vi "test_tcpclient.vi"() -> ()   [LabVIEW 2019]
panel:
  out "에러 출력":errorcluster
  out "길이":i32
  out "데이터 출력":string
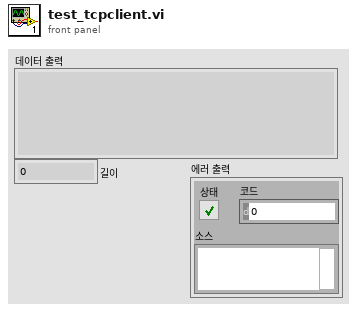
[diagram p1: front panel]
types:
  T1 = enum16{"Standard", "Buffered", "CRLF", "Immediate"}
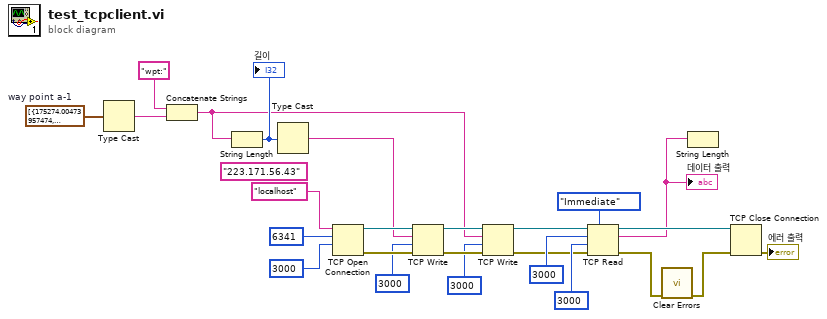
[diagram p0: block diagram]
diagram:
  (unwired) "223.171.56.43" ("Machine")
  w12 = cluster{"X":dbl, "Y":dbl}[] [{"X"=175274.00473957474, "Y"=530129.5157438602}, {"X"=175273.9994878598, "Y"=530129.5122022912}, {"X"=175273.88617325024, "Y"=530129.3515401008}, {"X"=175272.68065750896, "Y"=530127.4900123067}, {"X"=175272.6737370609, "Y"=530127.4862059783}, {"X"=175272.6643477536, "Y"=530127.4868430574}, {"X"=175272.65941880862, "Y"=530127.4861129179}, {"X"=175272.65828264618, "Y"=530127.4796280419}, {"X"=175272.65754210684, "Y"=530127.4685405197}, {"X"=175272.65886747447, "Y"=530127.4575323473}, {"X"=175275.24952781235, "Y"=530130.7235086206}, {"X"=175275.72679590562, "Y"=530131.2911066092}, {"X"=175276.22262929002, "Y"=530131.8883650973}, {"X"=175276.73046744007, "Y"=530132.5103790438}, {"X"=175277.2160084758, "Y"=530133.111474839}, {"X"=175277.7228783223, "Y"=530133.7379877474}, {"X"=175278.23467314534, "Y"=530134.3806933991}, {"X"=175278.74720273982, "Y"=530135.0409537714}, {"X"=175279.23987504462, "Y"=530135.6864052094}, {"X"=175280.91154517294, "Y"=530137.9295182931}, {"X"=175281.1794743994, "Y"=530138.2947289064}, {"X"=175281.44680856468, "Y"=530138.6510235704}, {"X"=175281.72463026966, "Y"=530139.0159308233}, {"X"=175282.0015102056, "Y"=530139.3688022257}, {"X"=175282.27945698082, "Y"=530139.7259944954}, {"X"=175282.55852373713, "Y"=530140.077914963}, {"X"=175282.8311483772, "Y"=530140.4203407691}, {"X"=175283.1033063822, "Y"=530140.7571409787}, {"X"=175283.37576432535, "Y"=530141.0959280683}, {"X"=175283.65336961742, "Y"=530141.4368242207}, {"X"=175283.92779126446, "Y"=530141.7740950054}, {"X"=175284.20385452232, "Y"=530142.1228424397}, {"X"=175284.47496994474, "Y"=530142.4665701878}, {"X"=175284.74596157094, "Y"=530142.8094792332}, {"X"=175285.0186950549, "Y"=530143.1588214315}, {"X"=175285.29130561682, "Y"=530143.5103371057}, {"X"=175285.56377946716, "Y"=530143.8635579381}, {"X"=175285.83036446967, "Y"=530144.2140548322}, {"X"=175286.10275126458, "Y"=530144.5741004624}, {"X"=175286.36828605848, "Y"=530144.9232298034}, {"X"=175286.63513163378, "Y"=530145.2764972708}, {"X"=175286.90739945296, "Y"=530145.6370704629}, {"X"=175287.1797670756, "Y"=530145.994256079}, {"X"=175287.4453014945, "Y"=530146.342989234}, {"X"=175287.70847312824, "Y"=530146.6934008283}, {"X"=175287.96834295726, "Y"=530147.0397678753}, {"X"=175288.21933206188, "Y"=530147.3826218339}, {"X"=175288.48230602973, "Y"=530147.73750566}, {"X"=175288.72661496594, "Y"=530148.0667469767}, {"X"=175288.97248932836, "Y"=530148.3963732349}, {"X"=175289.20325854485, "Y"=530148.6997193932}, {"X"=175289.4533325028, "Y"=530149.0263799197}, {"X"=175289.7170391103, "Y"=530149.3732351185}, {"X"=175289.94705338945, "Y"=530149.6807133132}, {"X"=175290.20929376624, "Y"=530150.0313974353}, {"X"=175290.44099765085, "Y"=530150.3384233768}, {"X"=175290.69107477734, "Y"=530150.6691870798}, {"X"=175290.93328572533, "Y"=530150.9923448646}, {"X"=175291.17306334805, "Y"=530151.3085965351}, {"X"=175291.42890964248, "Y"=530151.6447770832}, {"X"=175291.65563403358, "Y"=530151.9375893783}, {"X"=175291.89275191838, "Y"=530152.2404695762}, {"X"=175292.13425833316, "Y"=530152.5476597142}, {"X"=175292.38933595005, "Y"=530152.872240096}, {"X"=175292.63073491893, "Y"=530153.1751564976}, {"X"=175292.86438353983, "Y"=530153.4646986987}, {"X"=175293.08456251005, "Y"=530153.7373553545}, {"X"=175293.31933611992, "Y"=530154.0296189471}, {"X"=175293.5669353489, "Y"=530154.3429552813}, {"X"=175293.79013514795, "Y"=530154.6346082591}, {"X"=175293.99919699648, "Y"=530154.91043425}, {"X"=175294.23494612498, "Y"=530155.2225936522}, {"X"=175294.4618142799, "Y"=530155.528153441}, {"X"=175294.68670046306, "Y"=530155.8245694136}, {"X"=175294.8932319965, "Y"=530156.1005460762}, {"X"=175295.11416787718, "Y"=530156.3949848645}, {"X"=175295.3423867288, "Y"=530156.7029191155}, {"X"=175295.54093274107, "Y"=530156.9698773636}, {"X"=175295.77252229722, "Y"=530157.2770136676}, {"X"=175295.99228581943, "Y"=530157.568919915}, {"X"=175296.2108791497, "Y"=530157.857811919}, {"X"=175296.43384412082, "Y"=530158.1500960607}, {"X"=175296.65676498265, "Y"=530158.4451449964}, {"X"=175296.87656675442, "Y"=530158.733828123}, {"X"=175297.09878029334, "Y"=530159.0242344007}, {"X"=175297.3209100406, "Y"=530159.3192634964}, {"X"=175297.53946949937, "Y"=530159.61111341}, {"X"=175297.75729462548, "Y"=530159.9050631305}, {"X"=175297.97451755032, "Y"=530160.1915685921}, {"X"=175298.19257092883, "Y"=530160.4863322874}, {"X"=175298.40867646263, "Y"=530160.7769064768}, {"X"=175298.62256852756, "Y"=530161.0666281783}, {"X"=175298.83417822816, "Y"=530161.3513644824}, {"X"=175299.04778942713, "Y"=530161.6437706635}, {"X"=175299.47700209834, "Y"=530162.2207681962}, {"X"=175299.6962516632, "Y"=530162.5195904814}, {"X"=175299.91551021635, "Y"=530162.8160642846}, {"X"=175300.12963692454, "Y"=530163.1102869193}, {"X"=175300.34073252836, "Y"=530163.3991423576}, {"X"=175300.54502428067, "Y"=530163.6795729806}, {"X"=175300.7577223589, "Y"=530163.9708631652}, {"X"=175301.62616935943, "Y"=530165.1216823726}, {"X"=175302.5254593493, "Y"=530166.2863037863}, {"X"=175303.18527895535, "Y"=530167.1454968242}, {"X"=175303.62342696637, "Y"=530167.7159166778}, {"X"=175310.16097941765, "Y"=530176.5582115706}, {"X"=175311.60845001024, "Y"=530178.4564093163}, {"X"=175311.86030556855, "Y"=530178.7900606951}, {"X"=175312.11498075575, "Y"=530179.126174304}, {"X"=175312.62935982816, "Y"=530179.7996497159}, {"X"=175313.1375920335, "Y"=530180.4658226775}, {"X"=175313.3990189692, "Y"=530180.8068619235}, {"X"=175313.65881998377, "Y"=530181.146539741}, {"X"=175313.9177177645, "Y"=530181.4836165035}, {"X"=175314.17415214767, "Y"=530181.8221921967}, {"X"=175314.4395212584, "Y"=530182.1661021416}, {"X"=175314.7023115845, "Y"=530182.5087333805}, {"X"=175314.96900353231, "Y"=530182.8527781678}, {"X"=175315.23369983808, "Y"=530183.1956435259}, {"X"=175315.50157477424, "Y"=530183.5455604322}, {"X"=175315.77181018525, "Y"=530183.8960341865}, {"X"=175316.04542567665, "Y"=530184.247385859}, {"X"=175316.31955375904, "Y"=530184.6010511945}, {"X"=175316.84903058026, "Y"=530185.2820837225}, {"X"=175317.38129618068, "Y"=530185.9581514191}, {"X"=175317.91280706186, "Y"=530186.6327397156}, {"X"=175318.182062935, "Y"=530186.9719269531}, {"X"=175318.4552795316, "Y"=530187.3193476506}, {"X"=175319.0014159784, "Y"=530188.0142099282}, {"X"=175319.27483774978, "Y"=530188.3555402486}, {"X"=175319.5492389786, "Y"=530188.6974037511}, {"X"=175319.82539301965, "Y"=530189.0371189493}, {"X"=175320.09826249993, "Y"=530189.381323244}, {"X"=175320.37226519384, "Y"=530189.7271334985}, {"X"=175320.64393428696, "Y"=530190.0701027507}, {"X"=175320.9165769911, "Y"=530190.4185252064}, {"X"=175321.19328325742, "Y"=530190.7740132491}, {"X"=175321.45659139234, "Y"=530191.1140005968}, {"X"=175321.72941233087, "Y"=530191.461311584}, {"X"=175321.95251283867, "Y"=530191.7470001135}, {"X"=175322.16532464704, "Y"=530192.0220943327}, {"X"=175322.37067224752, "Y"=530192.2834971666}, {"X"=175322.56229437568, "Y"=530192.525027423}, {"X"=175322.73990554007, "Y"=530192.7495959902}, {"X"=175322.91422045446, "Y"=530192.9731865155}, {"X"=175323.08738154572, "Y"=530193.1905985337}, {"X"=175323.26548979027, "Y"=530193.4137283771}, {"X"=175323.43727148935, "Y"=530193.6328725251}, {"X"=175323.6096645412, "Y"=530193.8490726349}, {"X"=175323.80699074292, "Y"=530194.0964960849}, {"X"=175324.05614273442, "Y"=530194.4061107116}, {"X"=175324.31111888157, "Y"=530194.7286735323}, {"X"=175324.56704112957, "Y"=530195.0488684587}, {"X"=175324.83578187227, "Y"=530195.3871728731}, {"X"=175325.10834637488, "Y"=530195.7293249926}, {"X"=175325.38945439694, "Y"=530196.0823263065}, {"X"=175325.6722181846, "Y"=530196.4354126442}, {"X"=175325.95672967637, "Y"=530196.789425005}, {"X"=175326.24457830185, "Y"=530197.1504762445}, {"X"=175326.5286249899, "Y"=530197.506083755}, {"X"=175326.8080508342, "Y"=530197.8612032551}, {"X"=175327.0941640386, "Y"=530198.2291274525}, {"X"=175327.37333938808, "Y"=530198.5921299302}, {"X"=175327.65607127667, "Y"=530198.9641828123}, {"X"=175327.9397818841, "Y"=530199.334716748}, {"X"=175328.220501643, "Y"=530199.707514753}, {"X"=175328.5049111398, "Y"=530200.0795682647}, {"X"=175328.7949704538, "Y"=530200.4580267589}, {"X"=175329.07385205853, "Y"=530200.8277980806}, {"X"=175329.36379046313, "Y"=530201.2178327836}, {"X"=175329.66436532678, "Y"=530201.6225661638}, {"X"=175329.95547737126, "Y"=530202.0138116102}, {"X"=175330.25295598558, "Y"=530202.41901918}, {"X"=175330.53956022885, "Y"=530202.8108706116}, {"X"=175330.8419255085, "Y"=530203.2223300473}, {"X"=175331.13195201478, "Y"=530203.6179626812}, {"X"=175331.41571912347, "Y"=530204.010755906}, {"X"=175331.69713162916, "Y"=530204.4019945143}, {"X"=175331.98958687438, "Y"=530204.8024301422}, {"X"=175332.29121012747, "Y"=530205.2164278494}, {"X"=175332.5883215296, "Y"=530205.6155401273}, {"X"=175332.88285866773, "Y"=530206.0119009}, {"X"=175333.19089243043, "Y"=530206.4178487876}, {"X"=175333.49203705165, "Y"=530206.816168969}, {"X"=175333.79303850673, "Y"=530207.2110079534}, {"X"=175334.0893020318, "Y"=530207.5938922067}, {"X"=175334.3892063653, "Y"=530207.9855713523}, {"X"=175334.6769313669, "Y"=530208.3671245654}, {"X"=175334.95773330683, "Y"=530208.7361556918}, {"X"=175335.2323387888, "Y"=530209.0990575975}, {"X"=175335.51306748565, "Y"=530209.4603920867}, {"X"=175335.795338003, "Y"=530209.8291292372}, {"X"=175336.075867931, "Y"=530210.1873578326}, {"X"=175336.3589926412, "Y"=530210.5538095022}, {"X"=175336.63876707532, "Y"=530210.9195896094}, {"X"=175336.91411793797, "Y"=530211.2847901087}, {"X"=175337.18312003254, "Y"=530211.6465776593}, {"X"=175337.45269431596, "Y"=530212.0062625683}, {"X"=175337.7209553494, "Y"=530212.3690822715}, {"X"=175337.98944422093, "Y"=530212.7334773109}, {"X"=175338.25587926744, "Y"=530213.0979849639}, {"X"=175338.52868281276, "Y"=530213.4681063772}, {"X"=175338.8270715183, "Y"=530213.8710219278}, {"X"=175339.09987210427, "Y"=530214.2401578118}, {"X"=175339.36014116515, "Y"=530214.5890679677}, {"X"=175339.64015941726, "Y"=530214.9682290286}, {"X"=175339.91455805866, "Y"=530215.3392247901}, {"X"=175340.19204513606, "Y"=530215.716735207}, {"X"=175340.47255665058, "Y"=530216.0988848016}, {"X"=175340.7614513212, "Y"=530216.4867809507}, {"X"=175341.04350502143, "Y"=530216.8716629283}, {"X"=175341.33658991486, "Y"=530217.2774543162}, {"X"=175341.64410756333, "Y"=530217.7099119138}, {"X"=175341.923443017, "Y"=530218.1057118566}, {"X"=175342.22936364054, "Y"=530218.5355027524}, {"X"=175342.55279432627, "Y"=530218.9959007761}, {"X"=175342.853771716, "Y"=530219.4237218449}, {"X"=175343.1555258112, "Y"=530219.8539135159}, {"X"=175343.45287598448, "Y"=530220.2793768641}, {"X"=175343.75118908664, "Y"=530220.7039772415}, {"X"=175344.02648011563, "Y"=530221.0926561153}, {"X"=175344.31951030123, "Y"=530221.513938076}, {"X"=175344.61748993694, "Y"=530221.9456370183}, {"X"=175344.9215387921, "Y"=530222.3808929314}, {"X"=175345.2398094967, "Y"=530222.8343840825}, {"X"=175345.54070788863, "Y"=530223.261942445}, {"X"=175345.84672666568, "Y"=530223.6909019012}, {"X"=175346.14135953155, "Y"=530224.0964236386}, {"X"=175346.4818114266, "Y"=530224.5620700925}, {"X"=175346.79941728554, "Y"=530224.9956179837}, {"X"=175347.12591049456, "Y"=530225.4394857899}, {"X"=175347.44286325248, "Y"=530225.866352058}, {"X"=175347.7636738763, "Y"=530226.3017351214}, {"X"=175348.0793182589, "Y"=530226.7285975026}, {"X"=175348.3978399274, "Y"=530227.1606688595}, {"X"=175348.71413229345, "Y"=530227.5958266628}, {"X"=175349.03568725986, "Y"=530228.0346559128}, {"X"=175349.35136932984, "Y"=530228.4656335876}, {"X"=175349.63429763477, "Y"=530228.8502990768}, {"X"=175350.31202571455, "Y"=530229.7610748007}, {"X"=175350.9657620107, "Y"=530230.6222051637}, {"X"=175351.30501294706, "Y"=530231.0718611733}, {"X"=175352.98191093397, "Y"=530233.2849793285}, {"X"=175354.325094944, "Y"=530235.0392812236}, {"X"=175356.5139735839, "Y"=530237.9021652578}, {"X"=175357.11627366152, "Y"=530238.6805678556}, {"X"=175357.40969987572, "Y"=530239.059631174}, {"X"=175357.9977159878, "Y"=530239.8222138252}, {"X"=175358.58175825854, "Y"=530240.5853587184}, {"X"=175358.8800216713, "Y"=530240.9707595569}, {"X"=175359.17089952106, "Y"=530241.3456795723}, {"X"=175359.45570521321, "Y"=530241.7094456495}, {"X"=175359.7556257851, "Y"=530242.08400608}, {"X"=175360.0654265399, "Y"=530242.4592355064}, {"X"=175360.37610858618, "Y"=530242.8335511507}, {"X"=175360.6766469507, "Y"=530243.1926461258}, {"X"=175360.9757493711, "Y"=530243.5442038479}, {"X"=175361.28149900775, "Y"=530243.8940705459}, {"X"=175361.58179288538, "Y"=530244.242366232}, {"X"=175361.8795235083, "Y"=530244.5943442258}, {"X"=175362.1701690775, "Y"=530244.9335109157}, {"X"=175362.47002807373, "Y"=530245.2797391374}, {"X"=175362.75999962015, "Y"=530245.619241903}, {"X"=175363.04848654536, "Y"=530245.9575326451}, {"X"=175363.32893681235, "Y"=530246.291935935}, {"X"=175363.5833795738, "Y"=530246.5938537038}, {"X"=175363.8139917913, "Y"=530246.8664914699}, {"X"=175364.051439322, "Y"=530247.149266535}, {"X"=175364.27875054546, "Y"=530247.4193158604}, {"X"=175364.48140306285, "Y"=530247.6667112568}, {"X"=175364.68130373914, "Y"=530247.9081936695}, {"X"=175364.87212307978, "Y"=530248.1351448188}, {"X"=175365.05830122996, "Y"=530248.3405561815}, {"X"=175365.24934642285, "Y"=530248.5335349937}, {"X"=175365.4586938402, "Y"=530248.7211780654}, {"X"=175365.68035351747, "Y"=530248.885941745}, {"X"=175365.90327231257, "Y"=530249.0346165324}, {"X"=175366.13637149328, "Y"=530249.1652904893}, {"X"=175366.37079705653, "Y"=530249.2714382051}, {"X"=175366.61827390923, "Y"=530249.3659272505}, {"X"=175366.86756814134, "Y"=530249.4425965978}, {"X"=175367.11207690288, "Y"=530249.5058751716}, {"X"=175367.3567533101, "Y"=530249.5650245816}, {"X"=175367.62133496685, "Y"=530249.629879967}, {"X"=175367.86905430927, "Y"=530249.6933355606}, {"X"=175368.1517549946, "Y"=530249.7661407787}, {"X"=175368.41413817744, "Y"=530249.8400324802}, {"X"=175368.67676292398, "Y"=530249.9249654686}, {"X"=175368.95770089532, "Y"=530250.0176168601}, {"X"=175369.22670276524, "Y"=530250.1089982273}, {"X"=175369.50063303096, "Y"=530250.2033583766}, {"X"=175369.77402096745, "Y"=530250.2964393551}, {"X"=175370.0421101817, "Y"=530250.3874249985}, {"X"=175370.29664589485, "Y"=530250.4816636177}, {"X"=175370.53368479141, "Y"=530250.5680904333}, {"X"=175370.78877829644, "Y"=530250.6574362741}, {"X"=175371.04713739155, "Y"=530250.7475893599}, {"X"=175371.29533503368, "Y"=530250.8288002849}, {"X"=175371.55924210517, "Y"=530250.9034323096}, {"X"=175371.81141736405, "Y"=530250.9751788629}, {"X"=175372.05235837863, "Y"=530251.0394492042}, {"X"=175372.29207432698, "Y"=530251.0964913194}, {"X"=175372.54753447103, "Y"=530251.1479322227}, {"X"=175372.80985884863, "Y"=530251.1964750472}, {"X"=175373.0779618144, "Y"=530251.240423805}, {"X"=175373.34660774906, "Y"=530251.2834664334}, {"X"=175373.6152436773, "Y"=530251.3234125947}, {"X"=175373.88194546604, "Y"=530251.3601902636}, {"X"=175374.1938507625, "Y"=530251.4006926748}, {"X"=175374.51872925175, "Y"=530251.4433166765}, {"X"=175374.79900635238, "Y"=530251.482146475}, {"X"=175375.13868270424, "Y"=530251.5259788403}, {"X"=175375.45358824547, "Y"=530251.5683248173}, {"X"=175375.82978955292, "Y"=530251.6141916682}, {"X"=175376.17793499245, "Y"=530251.6580746012}, {"X"=175376.5139992762, "Y"=530251.7055702066}, {"X"=175376.87018973782, "Y"=530251.7555936353}, {"X"=175377.24026591453, "Y"=530251.8047892973}, {"X"=175377.59636930356, "Y"=530251.8604399993}, {"X"=175377.96688510012, "Y"=530251.9082270975}, {"X"=175378.35741249754, "Y"=530251.9509165223}, {"X"=175378.67374899556, "Y"=530251.9738647275}, {"X"=175379.00524160772, "Y"=530251.975895192}, {"X"=175379.35247739623, "Y"=530251.9689682503}, {"X"=175379.7125607502, "Y"=530251.9581977867}, {"X"=175380.0933729456, "Y"=530251.9500654789}, {"X"=175380.45119064956, "Y"=530251.9423638212}, {"X"=175380.79150680685, "Y"=530251.9408800876}, {"X"=175381.1301878372, "Y"=530251.9403068274}, {"X"=175381.47107652182, "Y"=530251.9410356049}, {"X"=175381.81160542736, "Y"=530251.941713292}, {"X"=175382.1583224557, "Y"=530251.9436135975}, {"X"=175382.50416204456, "Y"=530251.9471435535}, {"X"=175382.85047314703, "Y"=530251.951369127}, {"X"=175383.20556531035, "Y"=530251.9538985235}, {"X"=175383.55283039506, "Y"=530251.9560181338}, {"X"=175383.89244492707, "Y"=530251.9614254886}, {"X"=175384.2278018331, "Y"=530251.9786764916}, {"X"=175384.56469375637, "Y"=530252.0103555985}, {"X"=175384.90371252302, "Y"=530252.051392338}, {"X"=175385.24706478935, "Y"=530252.099438415}, {"X"=175385.58792804737, "Y"=530252.1459935226}, {"X"=175385.9193890007, "Y"=530252.1932400188}, {"X"=175386.2604837821, "Y"=530252.2369021791}, {"X"=175386.5911148225, "Y"=530252.2775530318}, {"X"=175386.9222903062, "Y"=530252.3006465423}, {"X"=175387.28229401182, "Y"=530252.2929121043}, {"X"=175387.62466421502, "Y"=530252.2799721844}, {"X"=175387.93027813133, "Y"=530252.2646488417}, {"X"=175388.2409991896, "Y"=530252.2450208705}, {"X"=175388.56240209253, "Y"=530252.220650116}, {"X"=175388.92052526696, "Y"=530252.190338978}, {"X"=175389.23687064392, "Y"=530252.1678687864}, {"X"=175389.5753376039, "Y"=530252.1406143736}, {"X"=175389.8778530315, "Y"=530252.1153481143}, {"X"=175390.22718472683, "Y"=530252.089512334}, {"X"=175390.5630890984, "Y"=530252.0655584557}, {"X"=175390.8979634547, "Y"=530252.0428584341}, {"X"=175391.22960317053, "Y"=530252.0226429336}, {"X"=175391.55867739816, "Y"=530252.0038422944}, {"X"=175391.87951033696, "Y"=530251.9907639447}, {"X"=175392.2046095326, "Y"=530251.9799060859}, {"X"=175392.52962813876, "Y"=530251.968753254}, {"X"=175392.83001022547, "Y"=530251.9584021192}, {"X"=175393.14728301077, "Y"=530251.9506727168}, {"X"=175393.49708130673, "Y"=530251.9374026364}, {"X"=175393.82750725327, "Y"=530251.9267311599}, {"X"=175394.17059054173, "Y"=530251.9137949592}, {"X"=175394.4962388502, "Y"=530251.9011054165}, {"X"=175394.83817748734, "Y"=530251.8892968993}, {"X"=175395.1707083754, "Y"=530251.8805415569}, {"X"=175395.50018190366, "Y"=530251.874615377}, {"X"=175395.826819296, "Y"=530251.8750570489}, {"X"=175396.1583653206, "Y"=530251.8756751856}, {"X"=175396.5042830234, "Y"=530251.877458572}, {"X"=175396.8405475861, "Y"=530251.8822858657}, {"X"=175397.18239753207, "Y"=530251.8884995996}, {"X"=175397.50686157987, "Y"=530251.8956867978}, {"X"=175397.81604317346, "Y"=530251.9040510306}, {"X"=175398.4295024424, "Y"=530251.9020373435}, {"X"=175398.70534019003, "Y"=530251.8834735376}, {"X"=175398.99656782713, "Y"=530251.8608079262}, {"X"=175399.30757322672, "Y"=530251.8321375054}, {"X"=175399.6049048782, "Y"=530251.8016771716}, {"X"=175399.93269610187, "Y"=530251.7652727236}, {"X"=175400.25263059515, "Y"=530251.7277116233}, {"X"=175400.58998456638, "Y"=530251.686740851}, {"X"=175400.9279063112, "Y"=530251.6406464219}, {"X"=175401.27526716323, "Y"=530251.5958327602}, {"X"=175401.61223600793, "Y"=530251.5582338065}, {"X"=175401.9462553822, "Y"=530251.5348464095}, {"X"=175402.2982480789, "Y"=530251.5204725924}, {"X"=175402.64419659323, "Y"=530251.5128534149}, {"X"=175402.98677064007, "Y"=530251.5041509671}, {"X"=175403.32783964058, "Y"=530251.4963164325}, {"X"=175403.6796434534, "Y"=530251.4906012388}, {"X"=175404.0374824952, "Y"=530251.485324459}, {"X"=175404.73283554547, "Y"=530251.497987947}, {"X"=175405.44333194202, "Y"=530251.526324773}, {"X"=175405.78273774288, "Y"=530251.5408744316}, {"X"=175406.13260808703, "Y"=530251.5560026348}, {"X"=175406.84007820534, "Y"=530251.584189772}, {"X"=175407.21819518215, "Y"=530251.6017188046}, {"X"=175407.61685593953, "Y"=530251.6222140131}, {"X"=175408.01630098786, "Y"=530251.6416325923}, {"X"=175408.41382776093, "Y"=530251.6614641503}, {"X"=175408.80551302017, "Y"=530251.6828744787}, {"X"=175409.18886973435, "Y"=530251.7068475684}, {"X"=175409.5831748973, "Y"=530251.7272757728}, {"X"=175409.97421534616, "Y"=530251.7471941827}, {"X"=175410.3724366284, "Y"=530251.7664466639}, {"X"=175412.859882497, "Y"=530251.8016303764}, {"X"=175413.2918917442, "Y"=530251.7949316904}, {"X"=175413.71308979805, "Y"=530251.7872492936}, {"X"=175414.12900935306, "Y"=530251.7753028244}, {"X"=175415.85854146598, "Y"=530251.6858203384}, {"X"=175416.29044020732, "Y"=530251.6547917974}, {"X"=175417.58223410405, "Y"=530251.5570219693}, {"X"=175418.0143192921, "Y"=530251.5240274081}, {"X"=175419.74071979214, "Y"=530251.3542399728}, {"X"=175420.58187408207, "Y"=530251.2210568525}, {"X"=175421.8569027836, "Y"=530251.0132566964}, {"X"=175430.4214667419, "Y"=530249.9058980814}, {"X"=175434.9886332713, "Y"=530249.0412887661}, {"X"=175439.17077453557, "Y"=530248.2399495235}, {"X"=175440.32554478582, "Y"=530247.9882953187}, {"X"=175440.70893072494, "Y"=530247.8973494029}, {"X"=175441.44425972813, "Y"=530247.708410251}, {"X"=175442.51074655657, "Y"=530247.4062529192}, {"X"=175443.58120099697, "Y"=530247.1029309275}, {"X"=175444.74799694892, "Y"=530246.7786050664}, {"X"=175445.52227258962, "Y"=530246.5656788277}, {"X"=175445.89519918812, "Y"=530246.4617108132}, {"X"=175446.64006663952, "Y"=530246.2710016328}, {"X"=175447.56398738606, "Y"=530246.0934468561}, {"X"=175447.8627750396, "Y"=530246.0492128325}, {"X"=175448.4682387152, "Y"=530245.9726726192}, {"X"=175448.7696215642, "Y"=530245.9320069747}, {"X"=175449.06859093998, "Y"=530245.8998832443}, {"X"=175449.67792215856, "Y"=530245.847847441}, {"X"=175450.0131588634, "Y"=530245.8223230243}, {"X"=175450.34109198756, "Y"=530245.7966913233}, {"X"=175450.6775091883, "Y"=530245.772286645}, {"X"=175451.00768058727, "Y"=530245.748732713}, {"X"=175451.659518, "Y"=530245.7100337361}, {"X"=175452.61561360906, "Y"=530245.6690087137}, {"X"=175453.24432312453, "Y"=530245.6432288187}, {"X"=175453.86761783602, "Y"=530245.624079629}, {"X"=175454.1741683298, "Y"=530245.6180987543}, {"X"=175454.49004392038, "Y"=530245.6174100706}, {"X"=175454.79940776218, "Y"=530245.6105608199}, {"X"=175455.12652893428, "Y"=530245.6025285065}, {"X"=175455.45483065274, "Y"=530245.5911076693}, {"X"=175455.76785470033, "Y"=530245.5870267968}, {"X"=175456.01352716915, "Y"=530245.5864632318}, {"X"=175456.23549961802, "Y"=530245.5753201456}, {"X"=175456.52665672192, "Y"=530245.5393684035}, {"X"=175456.82133914743, "Y"=530245.4952388696}, {"X"=175457.1017481744, "Y"=530245.4508349348}, {"X"=175457.3938744554, "Y"=530245.4049671154}, {"X"=175457.67032476896, "Y"=530245.3568867572}, {"X"=175457.97007889877, "Y"=530245.3023973808}, {"X"=175458.29792968603, "Y"=530245.2390432307}, {"X"=175458.62109199335, "Y"=530245.171146883}, {"X"=175458.94155206456, "Y"=530245.1021386319}, {"X"=175459.27168731208, "Y"=530245.0297346817}, {"X"=175459.61034335403, "Y"=530244.9559783454}, {"X"=175459.96329148472, "Y"=530244.8770913724}, {"X"=175460.30554731173, "Y"=530244.8012068883}, {"X"=175460.6726466043, "Y"=530244.7183639382}, {"X"=175461.0406298928, "Y"=530244.6367203875}, {"X"=175461.4371189839, "Y"=530244.5464816841}, {"X"=175461.84406690823, "Y"=530244.4527584249}, {"X"=175462.2348577757, "Y"=530244.3610070973}, {"X"=175462.6342722095, "Y"=530244.2694180475}, {"X"=175463.00349406843, "Y"=530244.1812061308}, {"X"=175463.38297303577, "Y"=530244.0917011125}, {"X"=175463.74226989844, "Y"=530243.9966050428}, {"X"=175464.14710109856, "Y"=530243.8679486318}, {"X"=175464.63066545464, "Y"=530243.7023170985}, {"X"=175465.12056310903, "Y"=530243.5273075659}, {"X"=175465.6082063077, "Y"=530243.3507331172}, {"X"=175466.09741630737, "Y"=530243.1692729405}, {"X"=175467.0106324301, "Y"=530242.8351051018}, {"X"=175467.45195417793, "Y"=530242.680714028}, {"X"=175467.8861658626, "Y"=530242.5302782886}, {"X"=175468.3180530301, "Y"=530242.3812700104}, {"X"=175468.74990989163, "Y"=530242.2306814056}, {"X"=175469.17279131338, "Y"=530242.0852844401}, {"X"=175469.5885831221, "Y"=530241.9420580923}, {"X"=175470.0107290114, "Y"=530241.7989529679}, {"X"=175470.43755309616, "Y"=530241.6553691073}, {"X"=175470.87175821327, "Y"=530241.5074895497}, {"X"=175471.31237600787, "Y"=530241.3564547389}, {"X"=175471.75343231903, "Y"=530241.2027161574}, {"X"=175472.19730795163, "Y"=530241.0471180857}, {"X"=175472.63905792116, "Y"=530240.8894730329}, {"X"=175473.07440536987, "Y"=530240.7336048022}, {"X"=175473.51163086394, "Y"=530240.5777943465}, {"X"=175473.94527615982, "Y"=530240.4235337916}, {"X"=175474.37105481443, "Y"=530240.2725859563}, {"X"=175474.80628896813, "Y"=530240.114006762}, {"X"=175475.25310936404, "Y"=530239.9512671513}, {"X"=175475.69401572942, "Y"=530239.7916558456}, {"X"=175476.15162292225, "Y"=530239.626100008}, {"X"=175476.60052935034, "Y"=530239.4678781369}, {"X"=175477.04299482977, "Y"=530239.3082967348}, {"X"=175477.48849811737, "Y"=530239.1491692592}, {"X"=175477.9336419908, "Y"=530238.9922226259}, {"X"=175478.37073352473, "Y"=530238.8368845093}, {"X"=175478.82245926422, "Y"=530238.6770795983}, {"X"=175479.2586957227, "Y"=530238.5186086851}, {"X"=175479.6947979952, "Y"=530238.3614955463}, {"X"=175480.12627572345, "Y"=530238.2065335795}, {"X"=175480.55989064183, "Y"=530238.0530081852}, {"X"=175480.97519760276, "Y"=530237.9028927151}, {"X"=175481.40200211524, "Y"=530237.748578248}, {"X"=175481.8183349306, "Y"=530237.5981912276}, {"X"=175482.23984126345, "Y"=530237.4479866102}, {"X"=175482.65686859243, "Y"=530237.2985165556}, {"X"=175483.07476879138, "Y"=530237.14947126}, {"X"=175483.50104987144, "Y"=530237.002704369}, {"X"=175483.92780791287, "Y"=530236.8545620953}, {"X"=175484.36068535925, "Y"=530236.7059535184}, {"X"=175484.77265742247, "Y"=530236.558537204}, {"X"=175485.19331821118, "Y"=530236.4048003152}, {"X"=175485.61807475335, "Y"=530236.245283502}, {"X"=175486.03928725596, "Y"=530236.0920966389}, {"X"=175486.45702766735, "Y"=530235.9371519698}, {"X"=175486.87269471106, "Y"=530235.7831934057}, {"X"=175487.29451064064, "Y"=530235.624926122}, {"X"=175487.7485673696, "Y"=530235.4515768033}, {"X"=175488.13795176853, "Y"=530235.3037451968}, {"X"=175488.5717418214, "Y"=530235.1361344861}, {"X"=175488.96341737075, "Y"=530234.9866558309}, {"X"=175489.37180375512, "Y"=530234.8288986009}, {"X"=175489.77758989108, "Y"=530234.6724852836}, {"X"=175490.17174664314, "Y"=530234.515480117}, {"X"=175490.58644432723, "Y"=530234.3492806158}, {"X"=175490.96764872826, "Y"=530234.2035996104}, {"X"=175491.372763613, "Y"=530234.0550805483}, {"X"=175491.79695489965, "Y"=530233.9042037404}, {"X"=175492.2151916093, "Y"=530233.7583409946}, {"X"=175492.64287779023, "Y"=530233.613058774}, {"X"=175493.05356312305, "Y"=530233.4722958092}, {"X"=175493.46724817288, "Y"=530233.3319868835}, {"X"=175493.86973957453, "Y"=530233.1943888749}, {"X"=175494.28287960906, "Y"=530233.049752028}, {"X"=175494.71242570534, "Y"=530232.8995311394}, {"X"=175495.12190582545, "Y"=530232.7546287056}, {"X"=175495.5276785231, "Y"=530232.6159257299}, {"X"=175495.9226521889, "Y"=530232.4818980738}, {"X"=175496.33357401242, "Y"=530232.3465340419}, {"X"=175496.7487477128, "Y"=530232.2075804946}, {"X"=175497.17735412085, "Y"=530232.0640238628}, {"X"=175497.58693363328, "Y"=530231.9288280853}, {"X"=175498.00855488758, "Y"=530231.7904450408}, {"X"=175498.40681873666, "Y"=530231.6622656975}, {"X"=175498.78026703003, "Y"=530231.548171062}, {"X"=175499.1925274097, "Y"=530231.4221937654}, {"X"=175499.62757159752, "Y"=530231.2936936121}, {"X"=175500.04906201834, "Y"=530231.1713984619}, {"X"=175500.43343634548, "Y"=530231.0611852489}, {"X"=175500.86102837036, "Y"=530230.9447389753}, {"X"=175501.29507063387, "Y"=530230.826464755}, {"X"=175501.7200278985, "Y"=530230.7074424973}, {"X"=175502.13735444294, "Y"=530230.5933548512}, {"X"=175502.5272443058, "Y"=530230.4857637095}, {"X"=175502.97811175193, "Y"=530230.364359312}, {"X"=175503.39027674735, "Y"=530230.2541591503}, {"X"=175503.80172853576, "Y"=530230.1436015066}, {"X"=175504.21858345164, "Y"=530230.0293610783}, {"X"=175504.61499804643, "Y"=530229.9263068892}, {"X"=175505.0092105549, "Y"=530229.8250527031}, {"X"=175505.39240597453, "Y"=530229.722682106}, {"X"=175505.77912372863, "Y"=530229.6101837333}, {"X"=175506.16221079679, "Y"=530229.4820070475}, {"X"=175506.54574761237, "Y"=530229.3501199122}, {"X"=175506.92381209665, "Y"=530229.2155185717}, {"X"=175507.2989338515, "Y"=530229.0790457674}, {"X"=175507.98891297288, "Y"=530228.8033189632}, {"X"=175508.28119228935, "Y"=530228.6718179771}, {"X"=175508.5912823027, "Y"=530228.5162086375}, {"X"=175509.225762145, "Y"=530228.1749486147}, {"X"=175509.9064732331, "Y"=530227.7872521307}, {"X"=175510.9833677454, "Y"=530227.170000761}, {"X"=175511.71006254628, "Y"=530226.7731898756}, {"X"=175513.55740866452, "Y"=530225.7904321894}, {"X"=175515.0718300646, "Y"=530225.00554216}, {"X"=175524.49975927762, "Y"=530219.3888609402}, {"X"=175528.21062942958, "Y"=530216.7515999195}, {"X"=175528.64031136382, "Y"=530216.4430135005}, {"X"=175531.59913054394, "Y"=530214.339004885}, {"X"=175532.89349644864, "Y"=530213.4102595663}, {"X"=175533.32674837907, "Y"=530213.0974144042}, {"X"=175534.16852558497, "Y"=530212.4856253457}, {"X"=175535.4119367021, "Y"=530211.5769648099}, {"X"=175535.8341984955, "Y"=530211.2742793995}, {"X"=175536.26860544292, "Y"=530210.9643699204}, {"X"=175536.68113032845, "Y"=530210.6703199997}, {"X"=175537.0999171656, "Y"=530210.3736502698}, {"X"=175537.52680909313, "Y"=530210.0721800154}, {"X"=175538.36408891596, "Y"=530209.4861355155}, {"X"=175538.78743155586, "Y"=530209.1849553934}, {"X"=175539.20161869272, "Y"=530208.8873891438}, {"X"=175539.6204356516, "Y"=530208.5864209707}, {"X"=175540.0340033643, "Y"=530208.2884425953}, {"X"=175540.45193806596, "Y"=530207.981090917}, {"X"=175540.86534855887, "Y"=530207.6774927184}, {"X"=175541.28450172965, "Y"=530207.3754437538}, {"X"=175541.69387156313, "Y"=530207.0773756357}, {"X"=175542.11383838835, "Y"=530206.7733587717}, {"X"=175542.53307651286, "Y"=530206.4739766129}, {"X"=175542.94941201503, "Y"=530206.1746162851}, {"X"=175543.37474526584, "Y"=530205.8712885495}, {"X"=175543.80899826958, "Y"=530205.5630691258}, {"X"=175544.24047627157, "Y"=530205.2603449834}, {"X"=175544.6710387351, "Y"=530204.9577356371}, {"X"=175545.10411323467, "Y"=530204.6526739477}, {"X"=175545.53446320922, "Y"=530204.3518943159}, {"X"=175545.94945464435, "Y"=530204.062040683}, {"X"=175546.3678788517, "Y"=530203.7695721919}, {"X"=175546.78023400935, "Y"=530203.486604107}, {"X"=175547.2017285433, "Y"=530203.1959990114}, {"X"=175547.62373835946, "Y"=530202.906209287}, {"X"=175548.04739087677, "Y"=530202.6132328131}, {"X"=175548.4811543025, "Y"=530202.3216451951}, {"X"=175548.92006300323, "Y"=530202.0245076861}, {"X"=175549.35435757096, "Y"=530201.7318786217}, {"X"=175549.79596376684, "Y"=530201.4329974513}, {"X"=175550.22925958788, "Y"=530201.1386721598}, {"X"=175550.65689797842, "Y"=530200.8398230008}, {"X"=175551.07740395996, "Y"=530200.5430623878}, {"X"=175551.50286695504, "Y"=530200.2384683457}, {"X"=175551.9143534468, "Y"=530199.9397286315}, {"X"=175552.3344331564, "Y"=530199.6343834606}, {"X"=175552.75555635593, "Y"=530199.3278288415}, {"X"=175553.17578555795, "Y"=530199.0172425224}, {"X"=175553.5941678406, "Y"=530198.7057182427}, {"X"=175554.02188108984, "Y"=530198.387549727}, {"X"=175554.44394939567, "Y"=530198.072155734}, {"X"=175554.87182918983, "Y"=530197.7454874746}, {"X"=175555.30316562232, "Y"=530197.4113364511}, {"X"=175555.74206029117, "Y"=530197.0746883692}, {"X"=175556.18003027307, "Y"=530196.7359320619}, {"X"=175556.60741191078, "Y"=530196.406070065}, {"X"=175557.03726672585, "Y"=530196.078944432}, {"X"=175557.4699052193, "Y"=530195.7459306509}, {"X"=175557.91012511431, "Y"=530195.4071323447}, {"X"=175558.3639548209, "Y"=530195.0612500014}, {"X"=175558.8194419781, "Y"=530194.71661587}, {"X"=175559.27039571086, "Y"=530194.3728884507}, {"X"=175559.73210858926, "Y"=530194.0286734558}, {"X"=175560.19752657512, "Y"=530193.6834876306}, {"X"=175560.66316681742, "Y"=530193.343415411}, {"X"=175561.11605628478, "Y"=530193.0194357058}, {"X"=175561.5641337951, "Y"=530192.6998651305}, {"X"=175562.0164112383, "Y"=530192.3725465877}, {"X"=175562.47725895798, "Y"=530192.0286450356}, {"X"=175562.9335391245, "Y"=530191.689127485}, {"X"=175563.39317344525, "Y"=530191.3437290017}, {"X"=175563.86363496457, "Y"=530190.9944543516}, {"X"=175564.32343549677, "Y"=530190.657408234}, {"X"=175564.75793670895, "Y"=530190.339323656}, {"X"=175565.20154090552, "Y"=530190.0132614688}, {"X"=175565.63567197032, "Y"=530189.6936763788}, {"X"=175566.0873603849, "Y"=530189.361708364}, {"X"=175566.53490329307, "Y"=530189.0360853422}, {"X"=175566.9805820106, "Y"=530188.7099783452}, {"X"=175567.4218713071, "Y"=530188.3810129929}, {"X"=175567.83879722763, "Y"=530188.0748421057}, {"X"=175568.28258719476, "Y"=530187.7458850304}, {"X"=175568.6779892812, "Y"=530187.4572462565}, {"X"=175569.13956524525, "Y"=530187.1177502025}, {"X"=175569.6352696651, "Y"=530186.7524545647}, {"X"=175570.07112028025, "Y"=530186.4288936092}, {"X"=175570.52449640125, "Y"=530186.0935669127}, {"X"=175570.9676058182, "Y"=530185.7656596776}, {"X"=175571.4398260512, "Y"=530185.40570459}, {"X"=175571.88895405893, "Y"=530185.066440393}, {"X"=175572.31587117087, "Y"=530184.7427058831}, {"X"=175572.78109950066, "Y"=530184.3898566399}, {"X"=175573.1902022406, "Y"=530184.0817644054}, {"X"=175573.6077431043, "Y"=530183.763390227}, {"X"=175574.0288520743, "Y"=530183.444753709}, {"X"=175574.45540775417, "Y"=530183.1270169334}, {"X"=175574.88283287873, "Y"=530182.8088292578}, {"X"=175575.33217064993, "Y"=530182.4654703671}, {"X"=175575.75112801587, "Y"=530182.1455683218}, {"X"=175576.16064843503, "Y"=530181.8293752683}, {"X"=175576.54712169807, "Y"=530181.5296033245}, {"X"=175576.98665616798, "Y"=530181.1967136014}, {"X"=175577.40578206035, "Y"=530180.8756324806}, {"X"=175577.79065536213, "Y"=530180.5818174423}, {"X"=175578.19222401528, "Y"=530180.2698030254}, {"X"=175578.56350140946, "Y"=530179.9866024712}, {"X"=175578.93215385434, "Y"=530179.6993286478}, {"X"=175579.29288462963, "Y"=530179.4162688048}, {"X"=175579.66397142026, "Y"=530179.1223742553}, {"X"=175580.04091095962, "Y"=530178.8170621587}, {"X"=175580.42300955596, "Y"=530178.5057528729}, {"X"=175580.7843972496, "Y"=530178.2192073312}, {"X"=175581.18055434595, "Y"=530177.9082343738}, {"X"=175581.5945580877, "Y"=530177.583829971}, {"X"=175582.01460639885, "Y"=530177.2572747867}, {"X"=175582.41097658096, "Y"=530176.956146826}, {"X"=175582.82576585156, "Y"=530176.6386301931}, {"X"=175583.20366597772, "Y"=530176.3533950043}, {"X"=175584.36886844857, "Y"=530175.5018527556}, {"X"=175584.74432513939, "Y"=530175.2316023164}, {"X"=175585.13131702453, "Y"=530174.9502751174}, {"X"=175585.50329752336, "Y"=530174.6786730683}, {"X"=175585.87885687826, "Y"=530174.4074579162}, {"X"=175586.25149480737, "Y"=530174.1407528976}, {"X"=175586.62138888295, "Y"=530173.8744521285}, {"X"=175586.98837385437, "Y"=530173.6099045669}, {"X"=175587.35262022124, "Y"=530173.352414841}, {"X"=175587.714133752, "Y"=530173.0951595226}, {"X"=175594.54207249463, "Y"=530168.1563049688}, {"X"=175598.27679705565, "Y"=530165.5389801083}, {"X"=175598.65417680735, "Y"=530165.2866389271}, {"X"=175599.03282612964, "Y"=530165.0298179962}, {"X"=175599.41434345095, "Y"=530164.765943329}, {"X"=175599.78918700153, "Y"=530164.5034987862}, {"X"=175600.17388477665, "Y"=530164.2330900147}, {"X"=175600.5613198794, "Y"=530163.9548609742}, {"X"=175600.94483522154, "Y"=530163.678701071}, {"X"=175601.3095423691, "Y"=530163.4155103841}, {"X"=175601.66596235512, "Y"=530163.1505892077}, {"X"=175601.9993656967, "Y"=530162.8986195598}, {"X"=175602.32196887277, "Y"=530162.6500753878}, {"X"=175602.64640996503, "Y"=530162.3978477935}, {"X"=175602.96049722412, "Y"=530162.153259614}, {"X"=175603.2852696097, "Y"=530161.9004151055}, {"X"=175603.6018799357, "Y"=530161.6525899002}, {"X"=175603.9041268309, "Y"=530161.4164823296}, {"X"=175604.2101937069, "Y"=530161.1808264365}, {"X"=175604.52793999258, "Y"=530160.9325051736}, {"X"=175604.85952707593, "Y"=530160.6688052947}, {"X"=175605.1825142698, "Y"=530160.4145953947}, {"X"=175605.49124765268, "Y"=530160.1729385317}, {"X"=175605.8018082719, "Y"=530159.931528288}, {"X"=175606.1080863333, "Y"=530159.6917109878}, {"X"=175606.41194238773, "Y"=530159.4557475364}, {"X"=175606.7096609258, "Y"=530159.2243757292}, {"X"=175606.99107867217, "Y"=530159.001942567}, {"X"=175607.27211166229, "Y"=530158.7796981023}, {"X"=175607.54564652068, "Y"=530158.5602102147}, {"X"=175607.79497316614, "Y"=530158.3651587978}, {"X"=175608.05474532628, "Y"=530158.159266891}, {"X"=175608.31203427628, "Y"=530157.9581124557}, {"X"=175608.56926956205, "Y"=530157.7537395926}, {"X"=175608.85215261197, "Y"=530157.5295220069}, {"X"=175609.07239568335, "Y"=530157.3549580018}, {"X"=175609.31950791806, "Y"=530157.1586900253}, {"X"=175609.52485898716, "Y"=530156.994412362}, {"X"=175609.7358453562, "Y"=530156.8276676956}, {"X"=175609.9206616476, "Y"=530156.6772232897}, {"X"=175610.12657691378, "Y"=530156.5074535237}, {"X"=175610.29158704227, "Y"=530156.3731387629}]  # way point a-1
  n1 = Type Cast(x=w12) -> (*(type *) &x=w11:string)  [unwired: 1 out]
  n2 = Concatenate Strings("wpt:" ("문자열"), w11) -> (w4:string)
  n3 = String Length(string=w4) -> (length=w10:i32)
  "길이" <- w10
  n4 = Type Cast(x=w10) -> (*(type *) &x=w5:string)  [unwired: 1 out]
  n5 = TCP Open Connection(address="localhost" ("Machine"), remote port or service name=u16 6341 ("Port"), timeout ms (60000)=3000 ("타임아웃 ms (60000)")) -> (connection ID=w18:refnum<k5>, error out=w15:errorcluster)  [unwired: 1 in, 1 out]
  n6 = TCP Write(connection ID=w18, data in=w5, error in (no error)=w15, 9:3000 ("타임아웃 ms (25000)")) -> (connection ID out=w8:refnum<k5>, error out=w9:errorcluster)  [unwired: 1 out]
  n7 = TCP Write(connection ID=w8, data in=w4, error in (no error)=w9, 9:3000 ("타임아웃 ms (25000)")) -> (connection ID out=w7:refnum<k5>, error out=w6:errorcluster)  [unwired: 1 out]
  n8 = TCP Read(connection ID=w7, bytes to read=3000, error in (no error)=w6, 7:T1."Immediate" ("mode (standard)"), 9:3000 ("timeout ms (25000)")) -> (connection ID out=w19:refnum<k5>, data out=w2:string, error out=w20:errorcluster)
  "데이터 출력" <- w2
  n9 = call <vilib>:"Clear Errors.vi"("error in (no error)"=w20) -> ("error out"=w16:errorcluster)  [unwired: 5 in, 1 out]
  n10 = String Length(string=w2) -> ()  [unwired: 1 out]
  n11 = TCP Close Connection(connection ID=w19, error in (no error)=w16) -> (error out=→"에러 출력":errorcluster)  [unwired: 1 in, 1 out]
